vi "ESP_tcpTest_server.vi"() -> ()   [LabVIEW 2022 SP3]
uses:
  <vilib>/Platform/TimedLoop/XDataNode/timing_clust.ctl
  <vilib>/Platform/TimedLoop/XDataNode/nitl_modes.ctl
  <vilib>/Platform/TimedLoop/XDataNode/wakeup.ctl
  <vilib>/platform/TimedLoop/XDataNode/XDataNode.xnode
  <vilib>/Platform/TimedLoop/XDataNode/XDNodeRunTimeDep.lvlib
panel:
  out "bytes written 2":i32
  out "bytes written":i32
  in  "stop":bool
  in  "Thermometer":dbl(slide) scale=0.0..4096.0
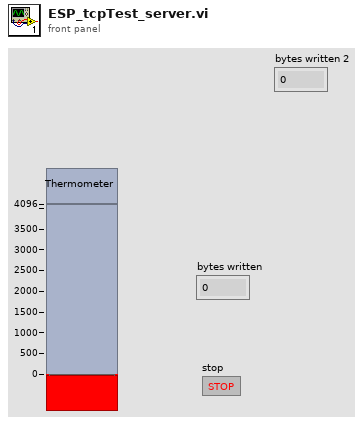
[diagram p1: front panel]
types:
  T1 = typedef "XDNodeRunTimeDep.lvlib/timing_clust.ctl" = cluster{"Expected End [f-1]":u64, "Actual End [f-1]":u64, "Finished Late? [f-1]":bool, "Expected End [i-1]":u64, "Actual End [i-1]":u64, "Finished Late? [i-1]":bool, "Expected Start [i]":u64, "Actual Start [i]":u64, "Expected Start [f]":u64, "Actual Start [f]":u64, "Source Name":string, "Structure Name":string, "Period":i64, "Deadline":i64, "Offset":i64, "Start":i64, "Priority":i32, "Timeout":i32, "Mode":T2, "Wakeup Reason":T3, "Error":errorcluster, "Source Type":string, "Secondary Source Type":string, "Global End Time":u64, "Global Start Time":u64, "Frame Duration":u64, "Iteration Duration":u64, "Assigned CPU":i32, "I/O Scan Engine Mode":u32}
  T2 = typedef "XDNodeRunTimeDep.lvlib/nitl_modes.ctl" = enum32{"No Change", "Process missed periods, maintain original phase", "Discard missed periods, maintain original phase", "Process missed periods, ignore original phase", "Discard missed periods, ignore original phase"}
  T3 = typedef "XDNodeRunTimeDep.lvlib/wakeup.ctl" = enum32{"Normal", "Aborted", "Asynchronous wakeup", "Timing source error", "Timed loop error", "Timeout"}
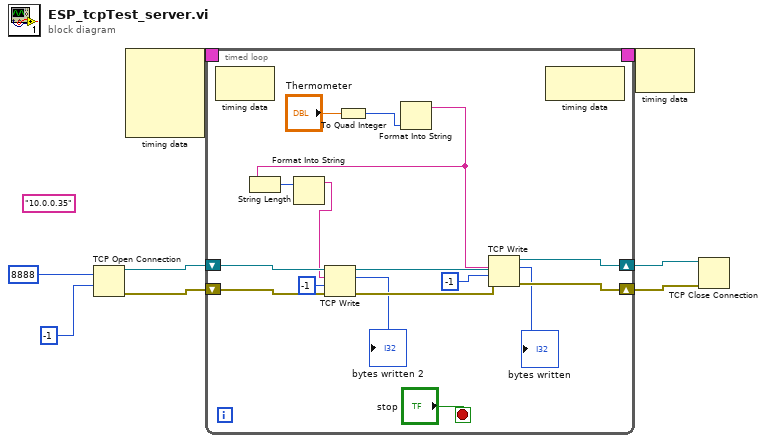
[diagram p0: block diagram]
diagram:
  (unwired) "10.0.0.35" ("address")
  n1 = TCP Open Connection(remote port or service name=u16 8888, timeout ms (60000)=-1) -> (connection ID=w5:refnum<k5>, error out=w8:errorcluster)  [unwired: 3 in]
  n2 = node-c288() -> (w2:T1)  [unwired: 4 in]
  n3 = timed-loop {
    timing: w2 -> [_]
    timing-out: [_] -> w1
    shift-right: [w22] -> w7
    shift-left: w8 -> [w24]
    shift-right: [w17] -> w4
    shift-left: w5 -> [w19]
    stop <- "stop" stop-if-true
    n4 = node-c288() -> ()  [unwired: 1 in, 1 out]
    n5 = To Quad Integer(1:"Thermometer") -> (0:w9:i64)
    n6 = Format Into String(w9) -> (resulting string=w14:string)  [unwired: 3 in, 1 out]
    n7 = String Length(string=w14) -> (length=w13:i32)
    n8 = Format Into String(w13) -> (resulting string=w12:string)  [unwired: 3 in, 1 out]
    n9 = TCP Write(connection ID=w19, data in=w12, error in (no error)=w24, 9:-1 ("timeout ms (25000)")) -> (connection ID out=w18:refnum<k5>, bytes written=→"bytes written 2":i32, error out=w23:errorcluster)
    n10 = TCP Write(connection ID=w18, data in=w14, error in (no error)=w23, 9:-1 ("timeout ms (25000)")) -> (connection ID out=w17:refnum<k5>, bytes written=→"bytes written":i32, error out=w22:errorcluster)
    n11 = node-c288() -> ()  [unwired: 1 in, 1 out]
  }
  n12 = node-c288(w1) -> ()  [unwired: 1 out]
  n13 = TCP Close Connection(connection ID=w4, error in (no error)=w7) -> ()  [unwired: 1 in, 2 out]
